vi "SCTL Sector Accumulation V3.vi"() -> (3 "New Data?":bool)   [LabVIEW 2013]
uses:
  <vilib>/rvi/FIFO/Fifo_Resource/nirvififoEmulationReadFpgaImpl.vi
  <vilib>/rvi/DataTransferAndStorage/Container/Common/niFpgaContainerGetUniqueNameForEmu.vi
  <vilib>/rvi/Memory/Memory_Emulation/nirvimemoryFastEmulationFpgaImpl.vi
  <instcachedir>/0/nirvimemoryFastEmulationFpgaImpl_5FBAB50466BC4C939F684F8805638BFC.lvgen/nirvimemoryFastEmulationFpgaImpl_5FBAB50466BC4C939F684F8805638BFC_011.vi
  <vilib>/rvi/Memory/Memory_Emulation/nirvimemoryFastEmulation.vi
  <vilib>/rvi/Memory/Memory_Emulation/nirvimemoryEmulation.vi
  <vilib>/rvi/DataTransferAndStorage/Container/XNode/niFpgaContainer.xnode
  <vilib>/rvi/FIFO/Fifo_Resource/nirvififoEmulationRead.vi
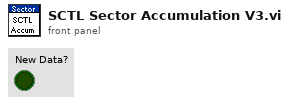
[diagram p1: front panel]
types:
  T1 = cluster{"Accumulated Intensity":u32, "Count":u16}
  T2 = cluster{"Accumulated Intensity":u32, "Count":u16}[]
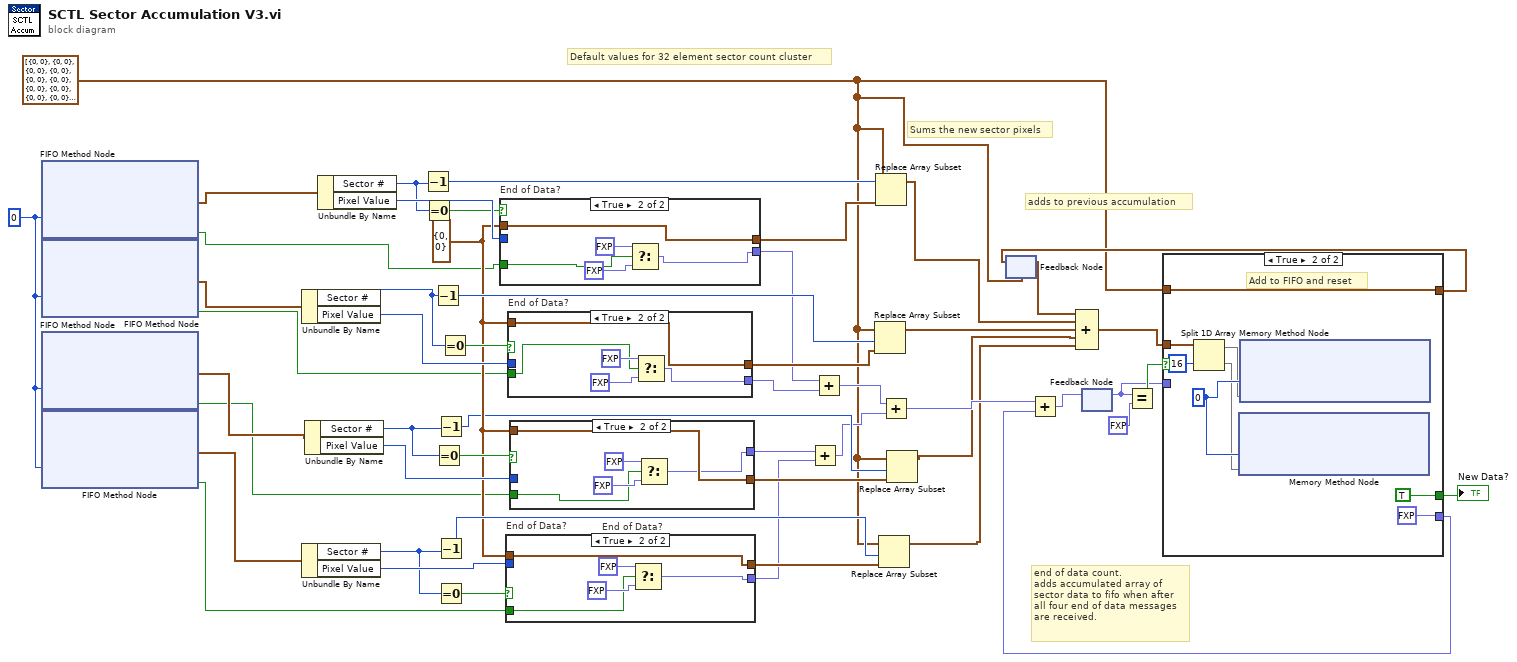
[diagram p0: block diagram]
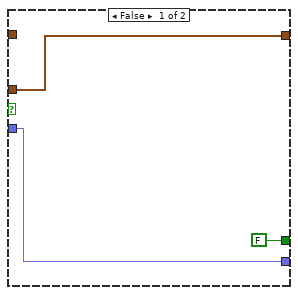
[diagram p2: hidden frame]
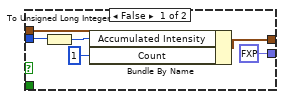
[diagram p3: hidden frame]
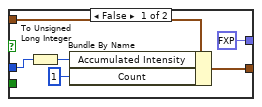
[diagram p4: hidden frame]
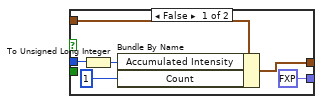
[diagram p5: hidden frame]
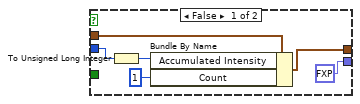
[diagram p6: hidden frame]
diagram:
  w27 = T1 {"Accumulated Intensity"=0, "Count"=0} ("Accumulated Sector Cluster")
  w1 = T2 [{"Accumulated Intensity"=0, "Count"=0}, {"Accumulated Intensity"=0, "Count"=0}, {"Accumulated Intensity"=0, "Count"=0}, {"Accumulated Intensity"=0, "Count"=0}, {"Accumulated Intensity"=0, "Count"=0}, {"Accumulated Intensity"=0, "Count"=0}, {"Accumulated Intensity"=0, "Count"=0}, {"Accumulated Intensity"=0, "Count"=0}, {"Accumulated Intensity"=0, "Count"=0}, {"Accumulated Intensity"=0, "Count"=0}, {"Accumulated Intensity"=0, "Count"=0}, {"Accumulated Intensity"=0, "Count"=0}, {"Accumulated Intensity"=0, "Count"=0}, {"Accumulated Intensity"=0, "Count"=0}, {"Accumulated Intensity"=0, "Count"=0}, {"Accumulated Intensity"=0, "Count"=0}, {"Accumulated Intensity"=0, "Count"=0}, {"Accumulated Intensity"=0, "Count"=0}, {"Accumulated Intensity"=0, "Count"=0}, {"Accumulated Intensity"=0, "Count"=0}, {"Accumulated Intensity"=0, "Count"=0}, {"Accumulated Intensity"=0, "Count"=0}, {"Accumulated Intensity"=0, "Count"=0}, {"Accumulated Intensity"=0, "Count"=0}, {"Accumulated Intensity"=0, "Count"=0}, {"Accumulated Intensity"=0, "Count"=0}, {"Accumulated Intensity"=0, "Count"=0}, {"Accumulated Intensity"=0, "Count"=0}, {"Accumulated Intensity"=0, "Count"=0}, {"Accumulated Intensity"=0, "Count"=0}, {"Accumulated Intensity"=0, "Count"=0}, {"Accumulated Intensity"=0, "Count"=0}] ("Data")
  w51 = 0 ("Timeout")
  # "end of data count.\nadds accumulated array of\nsector data to fifo when after\nall four end of data messages\nare received."
  # "adds to previous accumulation"
  # "Sums the new sector pixels"
  # "Default values for 32 element sector count cluster"
  n1 = xnode ("FIFO Method Node")("Timeout"=w51) -> ("Element"=w22:cluster{"Sector #":u8, "Pixel Value":u8}, "Timed Out?"=w18:bool)  [unwired: 1 in, 1 out]
  n2 = xnode ("FIFO Method Node")("Timeout"=w51) -> ("Element"=w21:cluster{"Sector #":u8, "Pixel Value":u8}, "Timed Out?"=w17:bool)  [unwired: 1 in, 1 out]
  n3 = xnode ("FIFO Method Node")("Timeout"=w51) -> ("Element"=w20:cluster{"Sector #":u8, "Pixel Value":u8}, "Timed Out?"=w16:bool)  [unwired: 1 in, 1 out]
  n4 = xnode ("FIFO Method Node")("Timeout"=w51) -> ("Element"=w19:cluster{"Sector #":u8, "Pixel Value":u8}, "Timed Out?"=w15:bool)  [unwired: 1 in, 1 out]
  n5 = Unbundle By Name(w21) -> ("Sector #"=w37:u8, "Pixel Value"=w47:u8)
  n6 = Unbundle By Name(w19) -> ("Sector #"=w33:u8, "Pixel Value"=w41:u8)
  n7 = Unbundle By Name(w20) -> ("Sector #"=w35:u8, "Pixel Value"=w44:u8)
  n8 = Unbundle By Name(w22) -> ("Sector #"=w39:u8, "Pixel Value"=w49:u8)
  n9 = Decrement(x=w39) -> (x-1=w50:u8)
  n10 = Equal To 0?(x=w39) -> (x = 0?=w38:bool)
  n11 = Decrement(x=w37) -> (x-1=w46:u8)
  n12 = Equal To 0?(x=w35) -> (x = 0?=w34:bool)
  n13 = Decrement(x=w35) -> (x-1=w25:u8)
  n14 = Decrement(x=w33) -> (x-1=w43:u8)
  n15 = Equal To 0?(x=w33) -> (x = 0?=w32:bool)
  n16 = Equal To 0?(x=w37) -> (x = 0?=w36:bool)
  n17 = case "End of Data?" shown="True" w38 {
    tunnel: w49 -> [w53 _]
    tunnel: [w57 w62] -> w48
    tunnel: w27 -> [w56 w62]
    tunnel: [fxp<+,1,1> 0.0 w58] -> w14
    tunnel: w18 -> [_ w61]
    frame False {
      n18 = To Unsigned Long Integer(number=w53) -> (unsigned 32bit integer=w52:u32)
      n19 = Bundle By Name(cluster=w56, "Accumulated Intensity"=w52, "Count"=u16 1) -> (w57:T1)
    }
    frame True {
      n20 = Select(t=fxp<+,1,1> 0.0, s=w61, f=fxp<+,1,1> 1.0) -> (s? t:f=w58:fxp<+,1,1>)
    }
  }
  n21 = case "End of Data?" shown="True" w32 {
    tunnel: [w68 w73] -> w42
    tunnel: w27 -> [w67 w73]
    tunnel: w41 -> [w64 _]
    tunnel: [fxp<+,1,1> 0.0 w69] -> w11
    tunnel: w15 -> [_ w70]
    frame False {
      n22 = To Unsigned Long Integer(number=w64) -> (unsigned 32bit integer=w63:u32)
      n23 = Bundle By Name(cluster=w67, "Accumulated Intensity"=w63, "Count"=u16 1) -> (w68:T1)
    }
    frame True {
      n24 = Select(t=fxp<+,1,1> 0.0, s=w70, f=fxp<+,1,1> 1.0) -> (s? t:f=w69:fxp<+,1,1>)
    }
  }
  n25 = case "End of Data?" shown="True" w36 {
    tunnel: w47 -> [w75 _]
    tunnel: w27 -> [w79 w84]
    tunnel: [w78 w84] -> w40
    tunnel: [fxp<+,1,1> 0.0 w80] -> w13
    tunnel: w17 -> [_ w81]
    frame False {
      n26 = To Unsigned Long Integer(number=w75) -> (unsigned 32bit integer=w74:u32)
      n27 = Bundle By Name(cluster=w79, "Accumulated Intensity"=w74, "Count"=u16 1) -> (w78:T1)
    }
    frame True {
      n28 = Select(t=fxp<+,1,1> 0.0, s=w81, f=fxp<+,1,1> 1.0) -> (s? t:f=w80:fxp<+,1,1>)
    }
  }
  n29 = case "End of Data?" shown="True" w34 {
    tunnel: [w90 w95] -> w45
    tunnel: w44 -> [w86 _]
    tunnel: w27 -> [w89 w95]
    tunnel: [fxp<+,1,1> 0.0 w91] -> w12
    tunnel: w16 -> [_ w92]
    frame False {
      n30 = To Unsigned Long Integer(number=w86) -> (unsigned 32bit integer=w85:u32)
      n31 = Bundle By Name(cluster=w89, "Accumulated Intensity"=w85, "Count"=u16 1) -> (w90:T1)
    }
    frame True {
      n32 = Select(t=fxp<+,1,1> 0.0, s=w92, f=fxp<+,1,1> 1.0) -> (s? t:f=w91:fxp<+,1,1>)
    }
  }
  n33 = Add(x=w12, y=w11) -> (x+y=w9:fxp<+,2,2>)
  n34 = Add(x=w14, y=w13) -> (x+y=w10:fxp<+,2,2>)
  n35 = Replace Array Subset(array=w1, new element=w40, index=w46) -> (w3:T2)
  n36 = Replace Array Subset(array=w1, new element=w48, index=w50) -> (w2:T2)
  n37 = Replace Array Subset(array=w1, new element=w42, index=w43) -> (w5:T2)
  n38 = Add(x=w10, y=w9) -> (x+y=w8:fxp<+,3,3>)
  n39 = Replace Array Subset(array=w1, new element=w45, index=w25) -> (w4:T2)
  n40 = feedback #1(w1) -> (w24:T2)
  n41 = Compound Arithmetic op=ADD(w24, w2, w3, w4, w5) -> (w23:T2)
  n42 = feedback #2() -> (w29:fxp<+,3,3>)  [unwired: 1 in]
  n43 = Equal?(x=w29, y=fxp<+,3,3> 4.0) -> (x = y?=w30:bool)
  n44 = case shown="True" w30 {
    tunnel: w23 -> [w98 w103]
    tunnel: [w96 fxp<+,3,3> 0.0] -> w7
    tunnel: w29 -> [w96 _]
    tunnel: [w98 w105] -> w28
    tunnel: w1 -> [_ w105]
    tunnel: [FALSE ("New Data?") TRUE ("New Data?")] -> w26
    frame False {
    }
    frame True {
      w104 = 0 ("Timeout")
      # "Add to FIFO and reset"
      n45 = Split 1D Array(array=w103, index=16) -> (first subarray=w101:T2, second subarray=w100:T2)
      n46 = xnode ("Memory Method Node")("Address"=w104, "Data"=w100) -> ()  [unwired: 1 in, 1 out]
      n47 = xnode ("Memory Method Node")("Address"=w104, "Data"=w101) -> ()  [unwired: 1 in, 1 out]
    }
  }
  "New Data?" <- w26
  n48 = feedback-in #1(w28) -> ()
  n49 = Add(x=w8, y=w7) -> (x+y=w6:fxp<+,3,3>)
  n50 = feedback-in #2(w6) -> ()
